vi "MatrixSwitchSingle.vi"(7 "Switch action":u16(ring) items=["Open", "Close"], 8 "error in (no error)":errorcluster, 9 "Matrix Y":i32=1 min=1 max=12 step=1, 10 "Matrix X":i32=1 min=1 max=12 step=1, 11 "Switching in":refnum<class "Switching.lvclass">) -> (0 "error out":errorcluster, 2 "command string":string, 3 "Switching out":refnum<class "Switching.lvclass">)   [LabVIEW 2018, in "Switching.lvclass"]
uses:
  Switching.lvclass
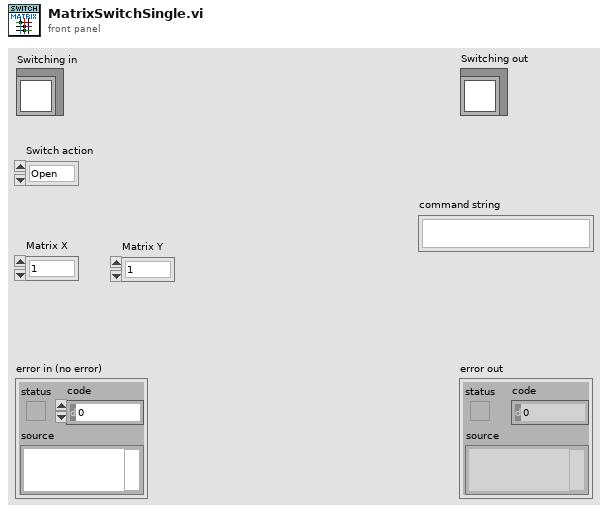
[diagram p1: front panel]
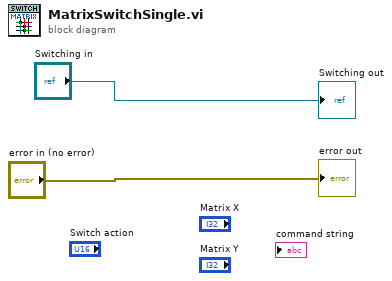
[diagram p0: block diagram]
diagram:
  "error out" <- "error in (no error)"
  "Switching out" <- "Switching in"
